vi "Configure DC Bias.vi"(7 "DC Bias State (F:Disable)":bool, 8 "error in (no error)":errorcluster, 9 "DC Bias Level (0.0 V)":dbl, 10 "DC Bias Type (0: Voltage)":u16(ring) items=["Voltage", "Current"], 11 "VISA resource name":refnum<visa-resource-name>) -> (0 "error out":errorcluster, 3 "VISA resource name out":refnum<visa-resource-name>)   [LabVIEW 2017, in "Agilent E4980.lvlib"]
doc: "Sets the DC bias state and level. You can set DC Bias level as voltage or current value."
uses:
  Agilent E4980.lvlib
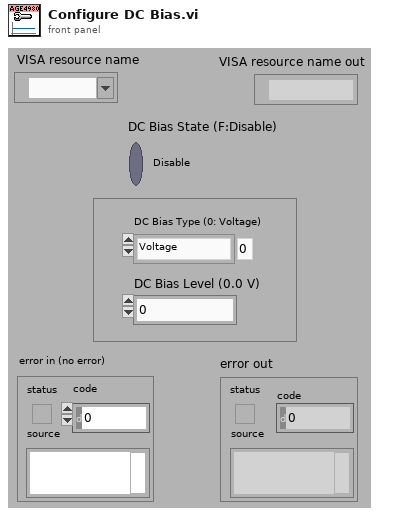
[diagram p1: front panel]
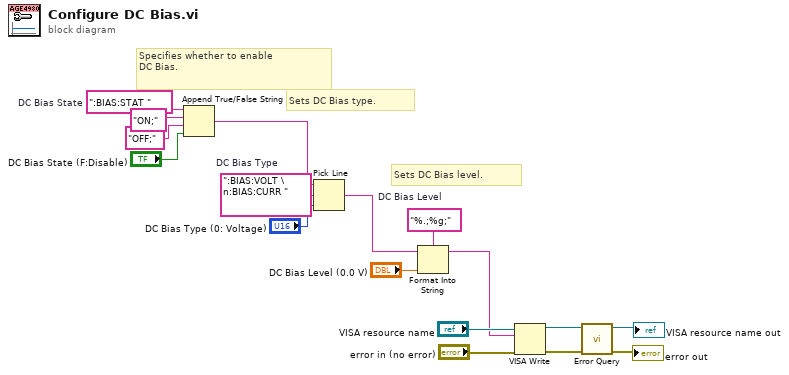
[diagram p0: block diagram]
diagram:
  w13 = "%.;%g;"  # DC Bias Level
  w16 = ":BIAS:VOLT \n:BIAS:CURR "  # DC Bias Type
  w5 = ":BIAS:STAT "  # DC Bias State
  # "Sets DC Bias level."
  # "Sets DC Bias type."
  # "Specifies whether to enable\nDC Bias."
  n1 = Append True/False String(1:"DC Bias State (F:Disable)", 2:"OFF;" ("f"), 3:"ON;", 4:w5) -> (0:w2:string)
  n2 = Pick Line(string ("")=w2, multi-line string=w16, line index="DC Bias Type (0: Voltage)") -> (output string=w15:string)
  n3 = Format Into String(format string=w13, initial string=w15, "DC Bias Level (0.0 V)") -> (resulting string=w10:string)  [unwired: 1 in, 1 out]
  n4 = VISA Write(VISA resource name="VISA resource name", write buffer=w10, error in (no error)="error in (no error)") -> (VISA resource name out=w9:refnum<visa-resource-name>, error out=w8:errorcluster)  [unwired: 1 out]
  n5 = call "Error Query.vi"("error in (no error)"=w8, "VISA resource name"=w9) -> ("error out"=→"error out":errorcluster, "VISA resource name out"=→"VISA resource name out":refnum<visa-resource-name>)  [unwired: 6 in, 2 out]
